vi "Test PyBaMM Wrapper.vi"() -> ()   [LabVIEW 2023]
uses:
  <vilib>/Python/Open Venv Python Session.vi
panel:
  out "terminal_voltages":dbl[](array[numeric])
  in  "time_step_s":dbl format="%#_13g"
  in  "current_A":dbl format="%#_13g"
  in  "number of simulation steps":i32
  in  "lower_voltage_cutoff":dbl=3.0 format="%#_13g"
  in  "upper_voltage_cutoff":dbl=4.2 format="%#_13g"
  in  "nominal_capacity_Ah":dbl=5.0 format="%#_13g"
  in  "C2":dbl=40000.0 format="%#_13g"
  in  "R2":dbl=0.0008 format="%#_13g"
  in  "C1":dbl=2500.0 format="%#_13g"
  in  "R1":dbl=0.001 format="%#_13g"
  in  "R0":dbl=0.0015 format="%#_13g"
  in  "num_rc_pairs":i32=1
  out "models":string[](array[string])
  out "chemistries":string[](array[string])
  in  "model_type":string="SPMe"
  in  "chemistry":string="Chen2020"
  out "simulation loaded":bool
  out "XY Graph":cluster{"X":dbl, "Y":dbl}[](graph)
  out "value":dbl[][](array[numeric])
  out "ocv_soc_profile":string
  out "profile loaded":bool
  in  "module path":path=path "C:/Repo/hps17k-panel/src/Python/hps17k-pybamm-wrapper.py"
  out "error out":errorcluster
  in  "venv path":path=path "C:/Repo/hps17k-panel/venv"
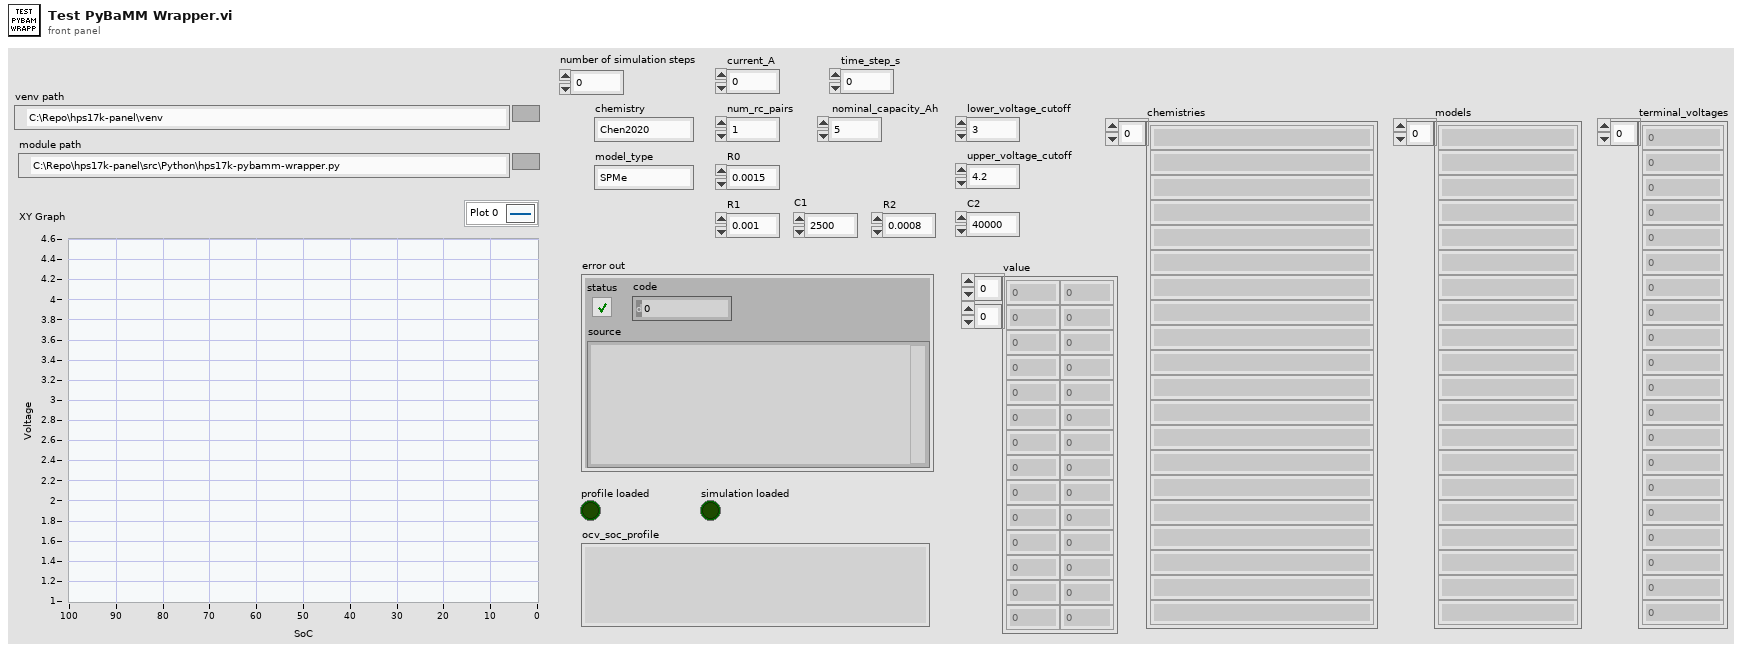
[diagram p1: front panel]
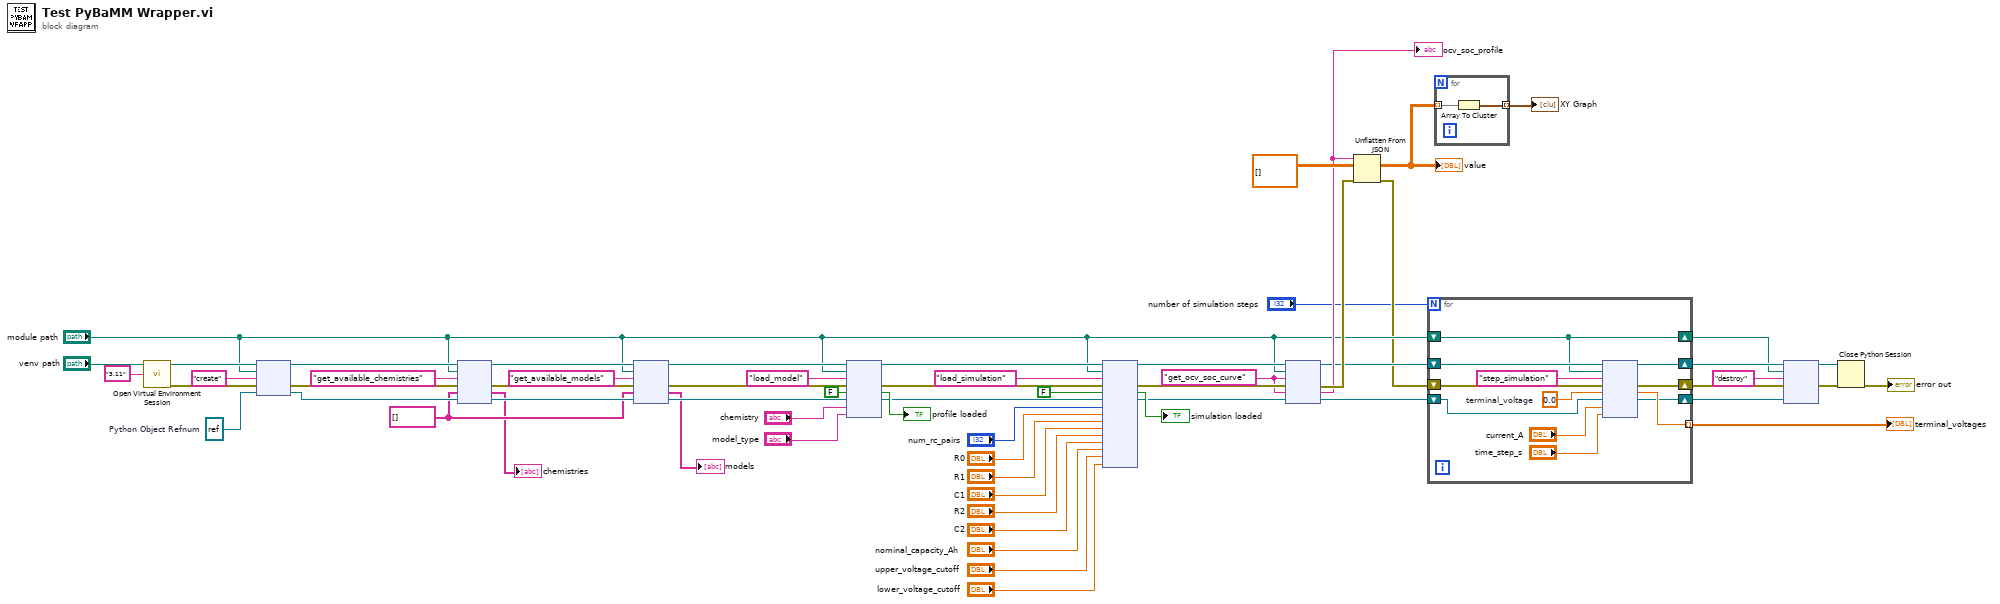
[diagram p0: block diagram]
diagram:
  w27 = string[] []
  w42 = "get_ocv_soc_curve" ("function name")
  w55 = refnum<k38> refnum  # Python Object Refnum
  n1 = call-poly <vilib>:"Open Virtual Environment Session.vi"("Python version"="3.11", "Env path"="venv path") -> ("error out"=w63:errorcluster, "session out"=w62:refnum<k35>)  [unwired: 8 in]
  n2 = node(w62, "module path", "create" ("function name"), w63, w55) -> (w34:refnum<k35>, w33:errorcluster, w32:refnum<k38>)  [unwired: 2 out]
  n3 = node(w34, "module path", "get_available_chemistries" ("function name"), w33, w27, w32) -> (w30:refnum<k35>, w29:errorcluster, →"chemistries":string[], w28:refnum<k38>)  [unwired: 2 out]
  n4 = node(w30, "module path", "get_available_models" ("function name"), w29, w27, w28) -> (w21:refnum<k35>, w24:errorcluster, →"models":string[], w26:refnum<k38>)  [unwired: 2 out]
  n5 = node(w21, "module path", "load_model" ("function name"), w24, FALSE, w26, "chemistry", "model_type") -> (w47:refnum<k35>, w48:errorcluster, →"profile loaded":bool, w46:refnum<k38>)  [unwired: 2 in, 2 out]
  n6 = node(w47, "module path", "load_simulation" ("function name"), w48, FALSE, w46, "num_rc_pairs", "R0", "R1", "C1", "R2", "C2", "nominal_capacity_Ah", "upper_voltage_cutoff", "lower_voltage_cutoff") -> (w44:refnum<k35>, w45:errorcluster, →"simulation loaded":bool, w43:refnum<k38>)  [unwired: 9 in, 2 out]
  n7 = node(w44, "module path", w42, w45, w42, w43) -> (w10:refnum<k35>, w39:errorcluster, w38:string, w2:refnum<k38>)  [unwired: 2 out]
  "ocv_soc_profile" <- w38
  n8 = Unflatten From JSON(JSON string=w38, type and defaults=dbl[][] [], error in (no error)=w39) -> (value=w4:dbl[][], error out=w9:errorcluster)  [unwired: 4 in]
  "value" <- w4
  n9 = for {
    N: "number of simulation steps" -> [_]
    shift-right: [w70] -> w7
    shift-left: "module path" -> [w70]
    shift-right: [w74] -> w8
    shift-left: w10 -> [w75]
    shift-right: [w73] -> w6
    shift-left: w9 -> [w72]
    tunnel: [w68] -> w3 mode=indexing
    shift-right: [w64] -> w1
    shift-left: w2 -> [w65]
    w69 = 0.0  # terminal_voltage
    n10 = node(w75, w70, "step_simulation" ("function name"), w72, w69, w65, "current_A", "time_step_s") -> (w74:refnum<k35>, w73:errorcluster, w68:dbl, w64:refnum<k38>)  [unwired: 2 in, 2 out]
  }
  "terminal_voltages" <- w3
  n11 = for {
    tunnel: w4 -> [w77] mode=indexing
    tunnel: [w76] -> w40 mode=indexing
    n12 = Array To Cluster(array=w77) -> (cluster=w76:cluster{"[0]":dbl, "[1]":dbl})
  }
  "XY Graph" <- w40
  n13 = node(w8, w7, "destroy" ("function name"), w6, w1) -> (w52:refnum<k35>, w53:errorcluster)  [unwired: 3 in, 2 out]
  n14 = Close Python Session(session in=w52, error in=w53) -> (11:→"error out":errorcluster)
